vi "PythonConverter_String.vi"(8 "error in":errorcluster, 11 "Name":string="TestAdd.vi") -> (0 "error out":errorcluster, 3 "PythonConverter out":refnum<class "PythonConverter_BD.lvclass">)   [LabVIEW 2014, in "PythonConverter_BD.lvclass"]
uses:
  PythonConverter_BD.lvclass
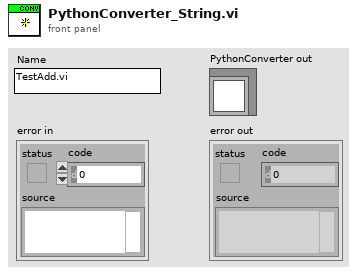
[diagram p1: front panel]
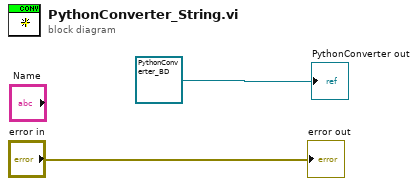
[diagram p0: block diagram]
diagram:
  "error out" <- "error in"
  "PythonConverter out" <- refnum<class "PythonConverter_BD.lvclass"> refnum ("PythonConverter in")
